vi "Read instr app PID.vi"(0 "Path":path=path "C:/ProgramData/Noffz/mmW_instr/BH_PID.json", 11 "error in":errorcluster) -> (4 "state":T1, 6 "watchdog timer":timestamp, 15 "error out":errorcluster)   [LabVIEW 2019, in "mmW_instr_app_API.lvlib"]
doc: "Reads file containing process status of Instrument Control app:\n\n- <b>state</b>: applicaiton state enum: Off, Initialization, Configuration, Running, Calibration\n- <b>watchdog timer</b>: time rvalue updated by app every 1 second, can be used to chech if app is running or stuck"
uses:
  mmW_instr_app_API.lvlib
  instr app state.ctl
  instr app PID content.ctl
  <vilib>/addons/_JKI.lib/Serialization/JSON/JKI JSON Serialization.lvlib
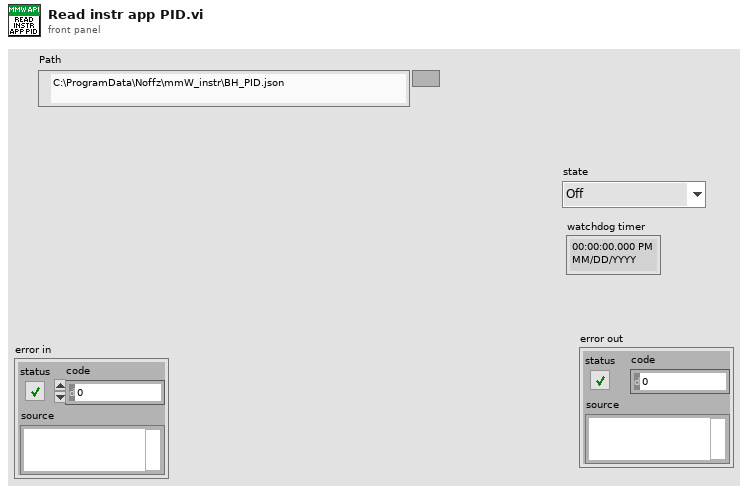
[diagram p1: front panel]
types:
  T1 = typedef "mmW_instr_app_API.lvlib/instr app state.ctl" = enum16{"Off", "Initialization", "Configuration", "Running", "Calibration"}
  T2 = typedef "mmW_instr_app_API.lvlib/instr app PID content.ctl" = cluster{"state":T1, "WD":dbl}
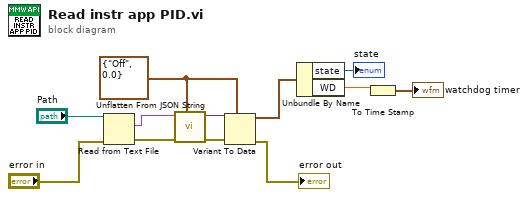
[diagram p0: block diagram]
diagram:
  w7 = T2 {"state"=enum."Off", "WD"=0.0} ("instr app PID")
  n1 = Read from Text File(file (use dialog)="Path", error in="error in") -> (text=w11:string, error out=w10:errorcluster)  [unwired: 2 in, 2 out]
  n2 = call <vilib>:"Unflatten From JSON String.vi"("Type and Defaults"=w7, "error in (no error)"=w10, "JSON String"=w11) -> ("error out"=w9:errorcluster, "Variant"=w8:variant)  [unwired: 7 in]
  n3 = Variant To Data(error in=w9, type=w7, Variant=w8) -> (data=w6:T2, error out=→"error out":errorcluster)
  n4 = Unbundle By Name(w6) -> ("state"=→"state":T1, "WD"=w3:dbl)
  n5 = To Time Stamp(1:w3) -> (0:→"watchdog timer":timestamp)
